vi "sv_Maximum Response (1 max type).vi"(8 "error in (no error)":errorcluster, 9 "maximum value type":i32(ring) items=["Maximax", "Initial positive", "Initial negative", "Initial absolute", "Residual positive", "Residual negative", "Residual absolute"], 10 "pulse duration [ms]":dbl=-1.0 format="%.2f", 11 "SDOF shock response":waveform(dbl)) -> (0 "error out":errorcluster, 1 "maximum time":dbl format="%.2f", 2 "maximum index":i32, 3 "maximum value":dbl format="%.2f")   [LabVIEW 2017, in "SoundVib_Transient.lvlib"]
doc: "Detects the values and locations of peaks for the single-degree-of-freedom (SDOF) vibration waveform, <B>SDOF vibration</B>."
uses:
  <vilib>/addons/Sound and Vibration/svt_Transients/SoundVib_Transient.lvlib
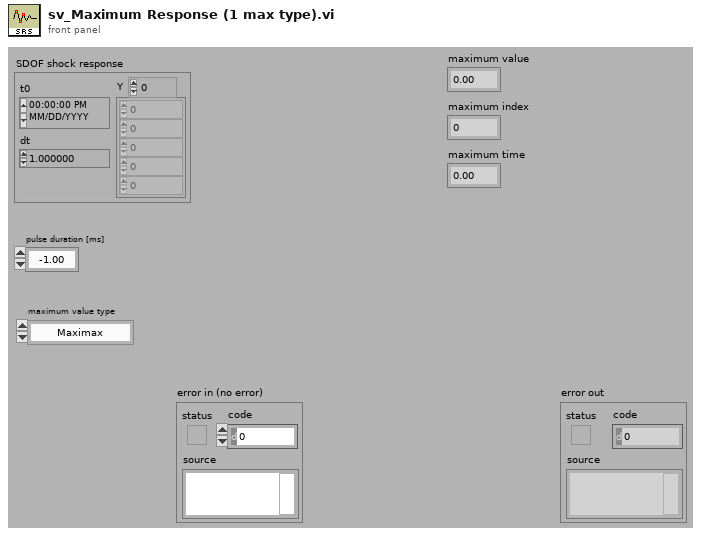
[diagram p1: front panel]
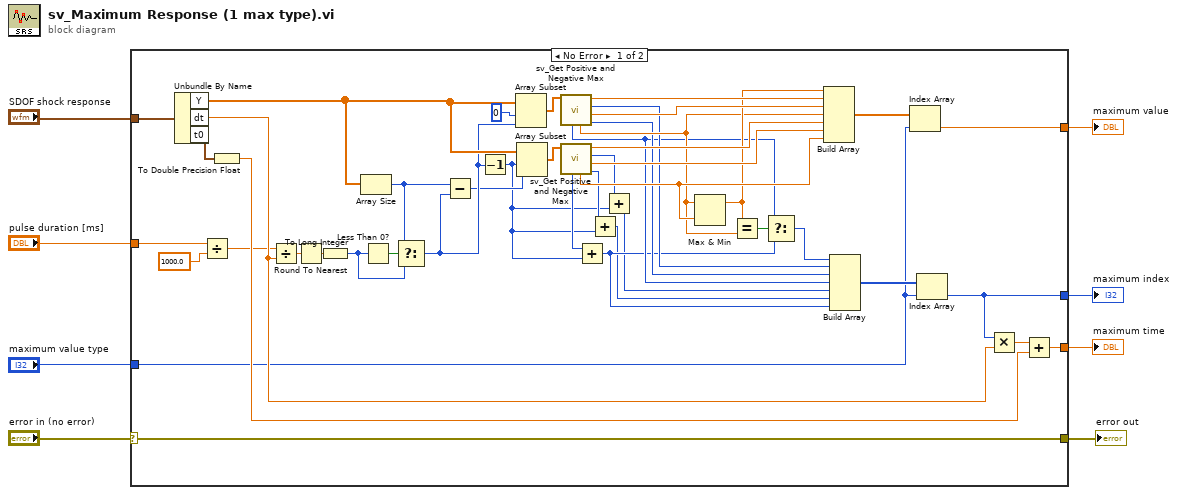
[diagram p0: block diagram]
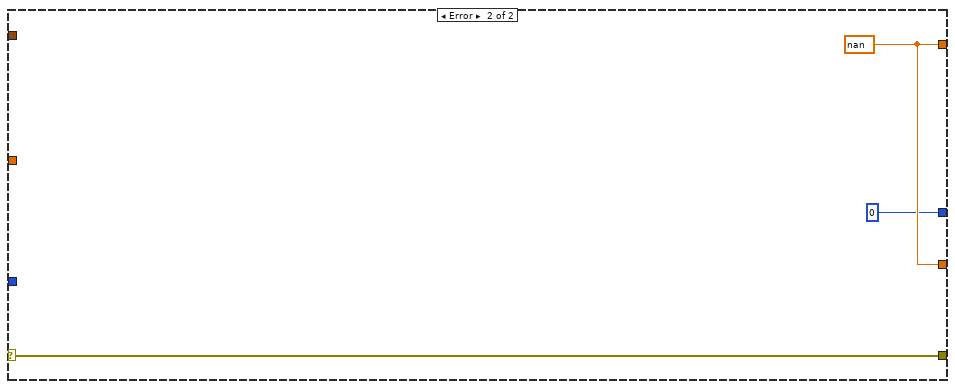
[diagram p2: hidden frame]
diagram:
  n1 = case shown="No Error" "error in (no error)" {
    selector: "error in (no error)" -> [w17 w56]
    tunnel: [w17 w56] -> w7
    tunnel: [w16 w55] -> w1
    tunnel: [w15 0] -> w2
    tunnel: [w14 w55] -> w3
    tunnel: "pulse duration [ms]" -> [w10 _]
    tunnel: "SDOF shock response" -> [w13 _]
    tunnel: "maximum value type" -> [w9 _]
    frame No Error {
      n2 = Unbundle By Name(w13) -> ("Y"=w51:dbl[], "dt"=w28:dbl, "t0"=w18:timestamp)
      n3 = Divide(x=w10, y=1000.0) -> (x/y=w12:dbl)
      n4 = To Double Precision Float(number=w18) -> (double precision float=w26:dbl)
      n5 = Divide(x=w12, y=w28) -> (x/y=w48:dbl)
      n6 = Round To Nearest(number=w48) -> (nearest integer value=w46:dbl)
      n7 = To Long Integer(number=w46) -> (32bit integer=w45:i32)
      n8 = Array Size(array=w51) -> (size(s)=w52:i32)
      n9 = Less Than 0?(x=w45) -> (x < 0?=w53:bool)
      n10 = Select(t=w52, s=w53, f=w45) -> (s? t:f=w50:i32)
      n11 = Subtract(x=w52, y=w50) -> (x-y=w49:i32)
      n12 = Decrement(x=w50) -> (x-1=w21:i32)
      n13 = Array Subset(array=w51, index=0 ("t0"), length=w50) -> (w44:dbl[])
      n14 = Array Subset(array=w51, index=w21, length=w49) -> (w43:dbl[])
      n15 = call <vilib>:"sv_Get Positive and Negative Max.vi"("data"=w44) -> ("negative index"=w31:i32, "negative max"=w39:dbl, "positive index"=w32:i32, "positive max"=w42:dbl, "absolute max"=w35:dbl, "abs max index"=w30:i32)  [unwired: 5 in]
      n16 = call <vilib>:"sv_Get Positive and Negative Max.vi"("data"=w43) -> ("negative index"=w23:i32, "negative max"=w37:dbl, "positive index"=w20:i32, "positive max"=w41:dbl, "absolute max"=w38:dbl, "abs max index"=w25:i32)  [unwired: 5 in]
      n17 = Add(x=w25, y=w21) -> (x+y=w24:i32)
      n18 = Add(x=w23, y=w21) -> (x+y=w22:i32)
      n19 = Add(x=w20, y=w21) -> (x+y=w19:i32)
      n20 = Max & Min(x=w35, y=w38) -> (max(x,y)=w36:dbl)  [unwired: 1 out]
      n21 = Equal?(x=w36, y=w35) -> (x = y?=w34:bool)
      n22 = Select(t=w30, s=w34, f=w24) -> (s? t:f=w33:i32)
      n23 = Build Array(w36, w42, w39, w35, w41, w37, w38) -> (w40:dbl[])
      n24 = Build Array(w33, w32, w31, w30, w19, w22, w24) -> (w29:i32[])
      n25 = Index Array(array=w40, index=w9) -> (element=w14:dbl)
      n26 = Index Array(array=w29, index=w9) -> (element=w15:i32)
      n27 = Multiply(x=w15, y=w28) -> (x*y=w27:dbl)
      n28 = Add(x=w27, y=w26) -> (x+y=w16:dbl)
    }
    frame Error {
      w55 = nan
    }
  }
  "error out" <- w7
  "maximum value" <- w3
  "maximum index" <- w2
  "maximum time" <- w1
